vi "Complex Kronecker Product.vi"(10 "B":T1, 11 "A":T1) -> (0 "error":i32, 3 "Kronecker Product":T1)   [LabVIEW 2024, in "NI_AALPro.lvlib"]
doc: "<p>Calculates the Kronecker product of the input matrices <strong>A</strong> and <strong>B</strong>. The data types you wire to the <strong>A</strong> and <strong>B</strong> inputs determine the polymorphic instance to use.</p>"
uses:
  NI_AALPro.lvlib
  ComplexMatrix.ctl
  <resource>/lvanlys.dll
  NI_Matrix.lvlib
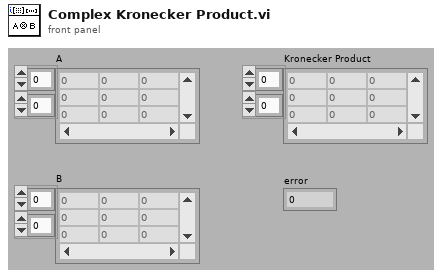
[diagram p1: front panel]
types:
  T1 = typedef "NI_Matrix.lvlib/ComplexMatrix.ctl" = cdb[][]
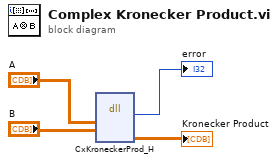
[diagram p0: block diagram]
diagram:
  n1 = dll-call lib="C:/Program Files (x86)/National Instruments/LabVIEW 2024/resource/lvanlys.*" fn="CxKroneckerProd_H"("A"="A", "B"="B") -> (→"error":i32, "Kronecker Product"=→"Kronecker Product":T1)  [unwired: 6 in, 2 out]
